vi "Log to file.vi"(6 "path":string, 9 "value":string, 10 "name":string, 11 "Byte Stream File in":refnum<file>) -> (3 "Byte Stream File out":refnum<file>)   [LabVIEW 2018]
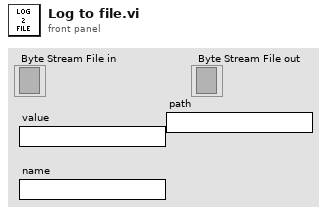
[diagram p1: front panel]
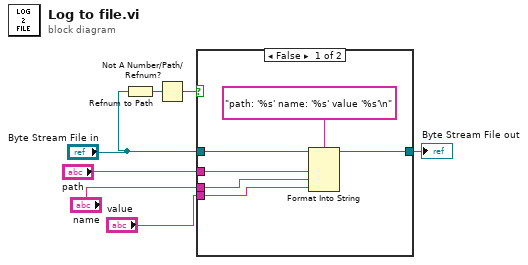
[diagram p0: block diagram]
diagram:
  n1 = Refnum to Path(1:"Byte Stream File in") -> (0:w2:path)
  n2 = Not A Number/Path/Refnum?(number/path/refnum=w2) -> (NaN/Path/Refnum?=w1:bool)
  n3 = case shown="False" w1 {
    tunnel: [w12 w14] -> w7
    tunnel: "Byte Stream File in" -> [w11 w14]
    tunnel: "path" -> [w10 _]
    tunnel: "name" -> [w9 _]
    tunnel: "value" -> [w8 _]
    frame False {
      n4 = Format Into String(format string="path: '%s' name: '%s' value '%s'\n", initial string=w11, w10, w9, w8) -> (resulting string=w12:refnum<file>)  [unwired: 1 in, 1 out]
    }
    frame True {
    }
  }
  "Byte Stream File out" <- w7
